vi "Update Tree Parents.vi"(8 "Error In":errorcluster, 11 "Tree Control In":refnum<vi>) -> (0 "Error Out":errorcluster, 3 "Tree Control Out":refnum<vi>)   [LabVIEW 2018, in "TraceTreeEditor.lvlib"]
uses:
  TraceTreeEditor.lvlib
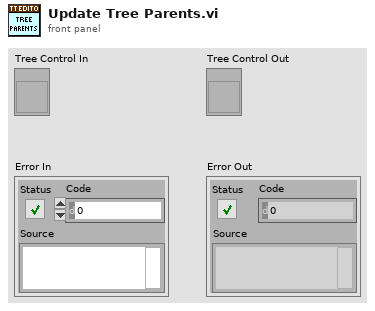
[diagram p1: front panel]
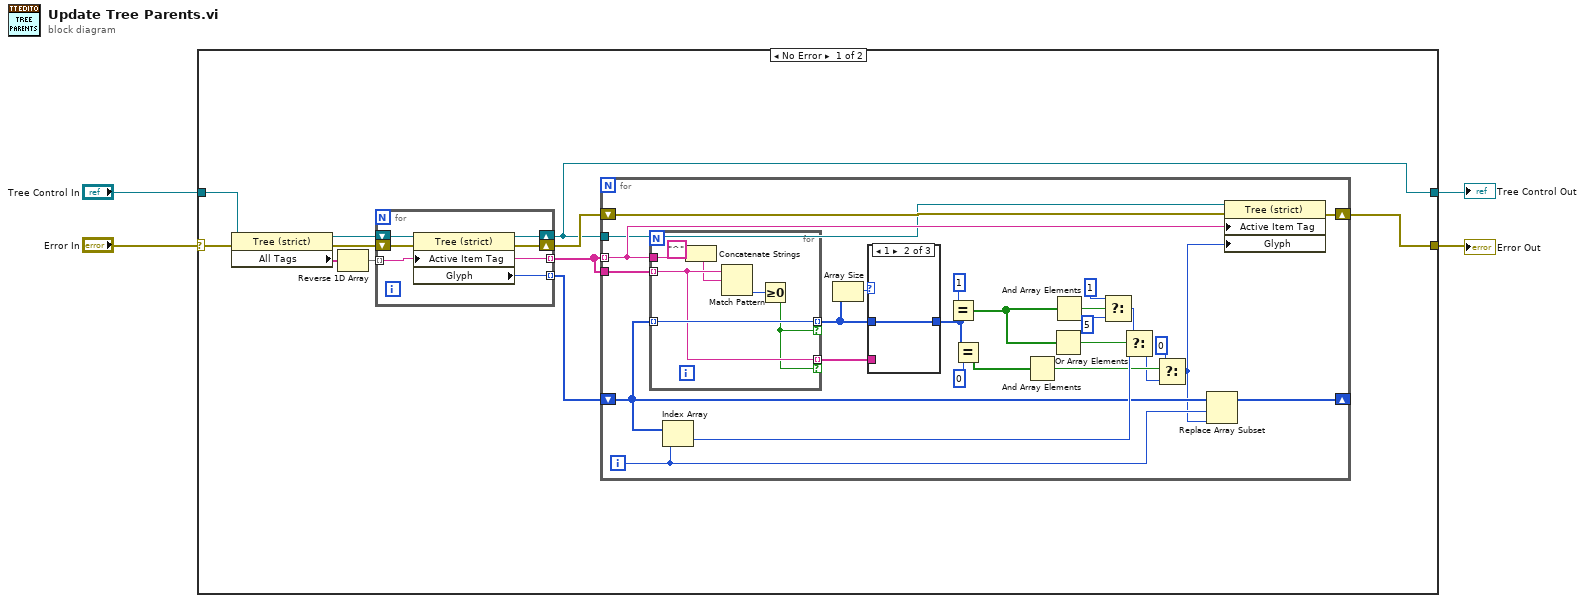
[diagram p0: block diagram]
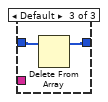
[diagram p3: hidden frame]
diagram:
  n1 = case shown="No Error" "Error In" {
    selector: "Error In" -> [w13 w60]
    tunnel: "Tree Control In" -> [w6 w59]
    tunnel: [w12 w60] -> w3
    tunnel: [w5 w59] -> w1
    frame No Error {
      n2 = property class="Tree (strict)"(reference=w6, error in=w13) -> (reference out=w8:refnum<vi>, error out=w15:errorcluster, "All Tags"=w7:string[])
      n3 = Reverse 1D Array(array=w7) -> (reversed array=w11:string[])
      n4 = for {
        tunnel: w11 -> [w55] mode=indexing
        tunnel: [w55] -> w9 mode=indexing
        tunnel: [w54] -> w10 mode=indexing
        shift-right: [w53] -> w5
        shift-left: w8 -> [w56]
        shift-right: [w57] -> w14
        shift-left: w15 -> [w58]
        n5 = property class="Tree (strict)"(reference=w56, error in=w58, "Active Item Tag"=w55) -> (reference out=w53:refnum<vi>, error out=w57:errorcluster, "Glyph"=w54:i32)
      }
      n6 = for {
        tunnel: w9 -> [w34]
        tunnel: w9 -> [w25] mode=indexing
        shift-right: [w28] -> _
        shift-left: w10 -> [w26]
        tunnel: w5 -> [w24]
        shift-right: [w40] -> w12
        shift-left: w14 -> [w41]
        i -> [w27]
        n7 = for {
          tunnel: w25 -> [w50]
          tunnel: w26 -> [w51] mode=indexing
          tunnel: w34 -> [w49] mode=indexing
          tunnel: [w51] -> w30 mode=indexing if=w48
          tunnel: [w49] -> w23 mode=indexing if=w48
          n8 = Concatenate Strings("^" ("string"), w50) -> (w47:string)
          n9 = Match Pattern(string=w49, regular expression=w47) -> (offset past match=w52:i32)  [unwired: 1 in, 3 out]
          n10 = Greater Or Equal To 0?(x=w52) -> (x >= 0?=w48:bool)
        }
        n11 = Index Array(array=w26, index=w27) -> (element=w29:i32)
        n12 = Array Size(array=w30) -> (size(s)=w31:i32)
        n13 = case shown="1" w31 {
          tunnel: w30 -> [w42 w43 w45]
          tunnel: [w42 w43 w44] -> w22
          tunnel: w23 -> [_ _ _]
          frame 0 {
          }
          frame 1 {
          }
          frame Default {
            n14 = Delete From Array(array=w45) -> (array with subset deleted=w44:i32[])  [unwired: 2 in, 1 out]
          }
        }
        n15 = Equal?(x=1, y=w22) -> (x = y?=w32:bool[])
        n16 = Equal?(x=w22, y=0) -> (x = y?=w20:bool[])
        n17 = And Array Elements(Boolean array=w20) -> (logical AND=w19:bool)
        n18 = Or Array Elements(Boolean array=w32) -> (logical OR=w36:bool)
        n19 = And Array Elements(Boolean array=w32) -> (logical AND=w39:bool)
        n20 = Select(t=1 ("y"), s=w39, f=5 ("y")) -> (s? t:f=w35:i32)
        n21 = Select(t=w35, s=w36, f=w29) -> (s? t:f=w18:i32)
        n22 = Select(t=0, s=w19, f=w18) -> (s? t:f=w17:i32)
        n23 = Replace Array Subset(array=w26, new element=w17, index=w27) -> (w28:i32[])
        n24 = property class="Tree (strict)"(reference=w24, error in=w41, "Active Item Tag"=w25, "Glyph"=w17) -> (error out=w40:errorcluster)  [unwired: 1 out]
      }
    }
    frame Error {
    }
  }
  "Error Out" <- w3
  "Tree Control Out" <- w1
